vi "[Generate Test Cases] Create directory.vi"(11 "Targets":T1(array[cluster])) -> (3 "Test Cases":refnum<class "TestCase.lvclass">[](array[class]))   [LabVIEW 2016, in "Tests.lvlib" / "[Test Suite] File Transfer Behavior.lvclass"]
uses:
  [Test Suite] File Transfer Behavior.lvclass
  <vilib>/addons/_JKI Toolkits/VI Tester/TestCase.llb/TestCase.lvclass
  [Test Case] Create directory/[Test Case] Create directory.lvclass
  classes/FTP/FTP.lvclass
  classes/WebDAV/WebDAV.lvclass
  classes/File Transfer Behavior/File Transfer Behavior.lvclass
  C:/GitHub/SystemManagementAndInformation/source/classes/File Transfer Behavior/File Transfer Behavior.lvclass
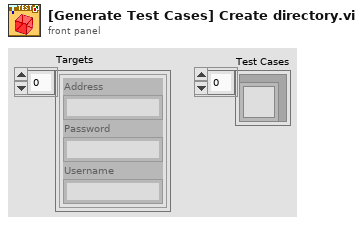
[diagram p1: front panel]
types:
  T1 = cluster{"Address":string, "Password":string, "Username":string}[]
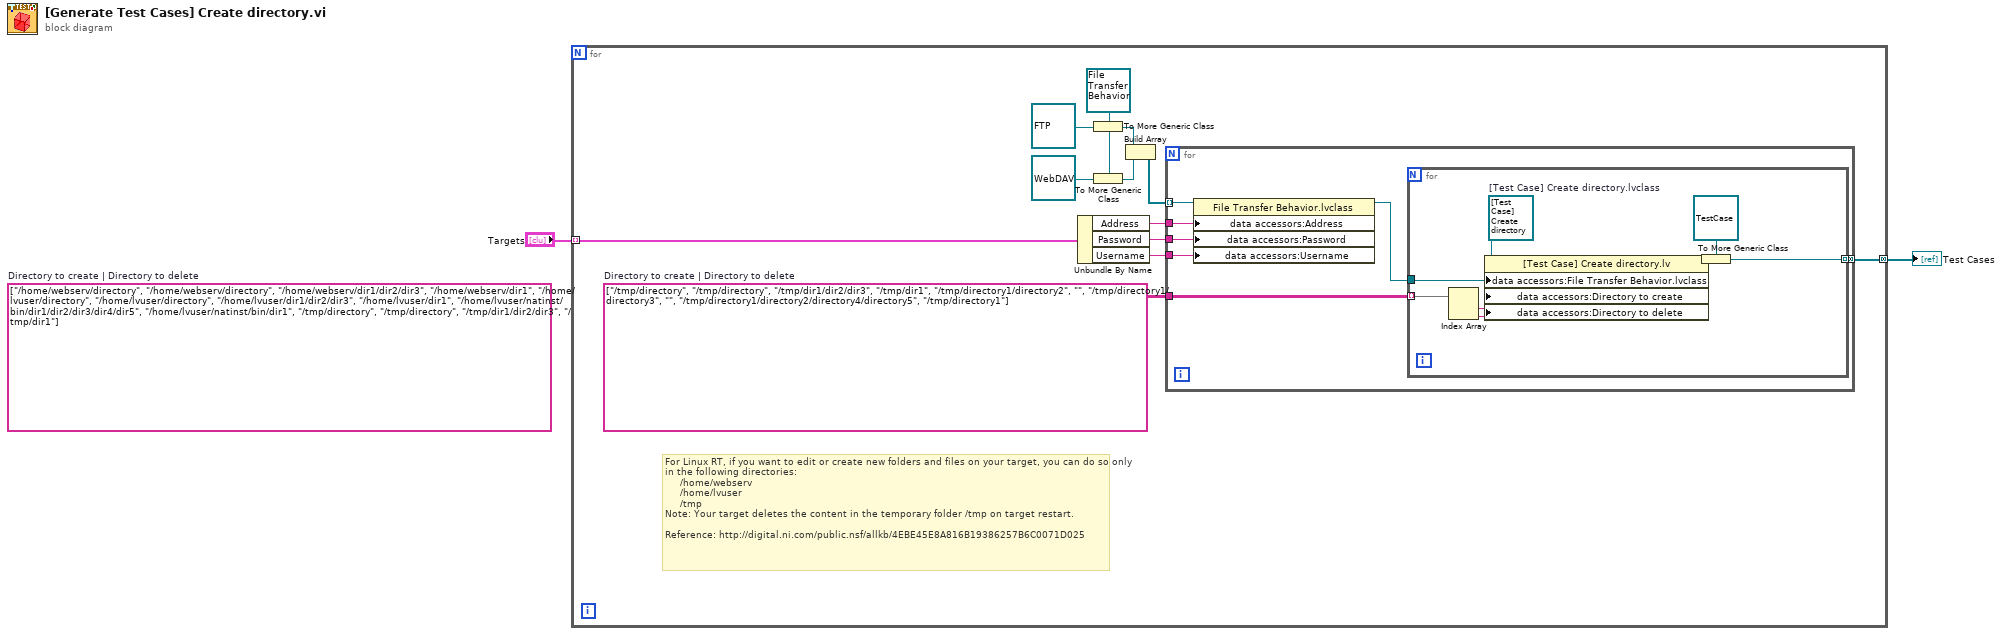
[diagram p0: block diagram]
diagram:
  (unwired) string[][] [["/home/webserv/directory", "/home/webserv/directory"], ["/home/webserv/dir1/dir2/dir3", "/home/webserv/dir1"], ["/home/lvuser/directory", "/home/lvuser/directory"], ["/home/lvuser/dir1/dir2/dir3", "/home/lvuser/dir1"], ["/home/lvuser/natinst/bin/dir1/dir2/dir3/dir4/dir5", "/home/lvuser/natinst/bin/dir1"], ["/tmp/directory", "/tmp/directory"], ["/tmp/dir1/dir2/dir3", "/tmp/dir1"]]  # Directory to create | Directory to delete
  n1 = for {
    tunnel: [w13] -> w2 mode=concatenating
    tunnel: "Targets" -> [w9] mode=indexing
    w8 = refnum<class "File Transfer Behavior.lvclass"> refnum ("RT Management.lvlib:File Transfer Behavior.lvclass")
    w14 = string[][] [["/tmp/directory", "/tmp/directory"], ["/tmp/dir1/dir2/dir3", "/tmp/dir1"], ["/tmp/directory1/directory2", ""], ["/tmp/directory1/directory3", ""], ["/tmp/directory1/directory2/directory4/directory5", "/tmp/directory1"]]  # Directory to create | Directory to delete
    # "For Linux RT, if you want to edit or create new folders and files on your target, you can do so only in the following directories:\n     /home/webserv\n     /home/lvuser\n     /tmp\nNote: Your target deletes the content in the temporary folder /tmp on target restart.\n\nReference: http://digital.ni.com/public.nsf/allkb/4EBE45E8A816B19386257B6C0071D025"
    n2 = Unbundle By Name(w9) -> ("Address"=w12:string, "Password"=w11:string, "Username"=w10:string)
    n3 = To More Generic Class(target class=w8, reference=refnum<class "FTP.lvclass"> refnum ("RT Management.lvlib:FTP.lvclass")) -> (generic class reference=w5:refnum<class "File Transfer Behavior.lvclass">)
    n4 = To More Generic Class(target class=w8, reference=refnum<class "WebDAV.lvclass"> refnum ("RT Management.lvlib:WebDAV.lvclass")) -> (generic class reference=w4:refnum<class "File Transfer Behavior.lvclass">)
    n5 = Build Array(w5, w4) -> (w3:refnum<class "File Transfer Behavior.lvclass">[])
    n6 = for {
      tunnel: w12 -> [w20]
      tunnel: w11 -> [w19]
      tunnel: w10 -> [w18]
      tunnel: w14 -> [w17]
      tunnel: [w16] -> w13 mode=concatenating
      tunnel: w3 -> [w15] mode=indexing
      n7 = property class="File Transfer Behavior.lvclass"(reference=w15, "data accessors:Address"=w20, "data accessors:Password"=w19, "data accessors:Username"=w18) -> (reference out=w21:refnum<class "File Transfer Behavior.lvclass">)  [unwired: 1 in, 1 out]
      n8 = for {
        tunnel: w21 -> [w28]
        tunnel: w17 -> [w24] mode=indexing
        tunnel: [w25] -> w16 mode=indexing
        w29 = refnum<class "[Test Case] Create directory.lvclass"> refnum  # [Test Case] Create directory.lvclass
        n9 = Index Array(array=w24) -> (element #1=w23:string, element #2=w22:string)  [unwired: 2 in]
        n10 = property class="[Test Case] Create directory.lv"(reference=w29, "data accessors:File Transfer Behavior.lvclass"=w28, "data accessors:Directory to create"=w23, "data accessors:Directory to delete"=w22) -> (reference out=w27:refnum<class "[Test Case] Create directory.lvclass">)  [unwired: 1 in, 1 out]
        n11 = To More Generic Class(target class=refnum<class "TestCase.lvclass"> refnum ("TestCase.lvclass"), reference=w27) -> (generic class reference=w25:refnum<class "TestCase.lvclass">)
      }
    }
  }
  "Test Cases" <- w2
